vi "Set Log File Producer Flag.vi"(8 "error in":errorcluster, 10 "log file producer":bool, 11 "custom device item in":T1 format="%.0x") -> (0 "error out":errorcluster, 3 "custom device item out":T1 format="%.0x")   [LabVIEW 2027, in "Embedded Data Logger Scripting.lvlib"]
uses:
  Embedded Data Logger Scripting.lvlib
  <vilib>/NI VeriStand/Custom Device API/Custom Device Item Ref.ctl
  <vilib>/NI VeriStand/Custom Device API/Custom Device API.lvlib
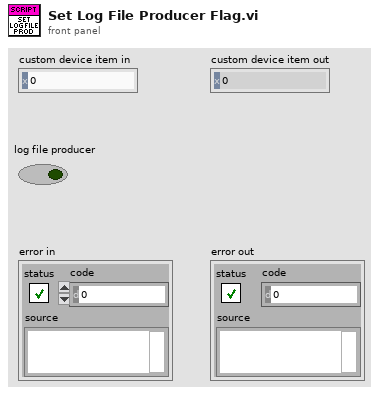
[diagram p1: front panel]
types:
  T1 = typedef "Custom Device API.lvlib/Custom Device Item Ref.ctl" = u64
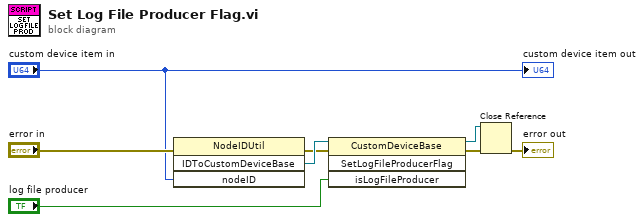
[diagram p0: block diagram]
diagram:
  n1 = invoke class="NodeIDUtil" method="IDToCustomDeviceBase"(error in="error in", "nodeID"="custom device item in") -> (error out=w3:errorcluster, "IDToCustomDeviceBase"=w8:refnum<k39>)  [unwired: 2 in, 2 out]
  n2 = invoke class="CustomDeviceBase" method="SetLogFileProducerFlag"(reference=w8, error in=w3, "isLogFileProducer"="log file producer") -> (reference out=w4:refnum<k39>, error out=w5:errorcluster)  [unwired: 1 in, 2 out]
  n3 = Close Reference(reference=w4, error in (no error)=w5) -> (error out=→"error out":errorcluster)
  "custom device item out" <- "custom device item in"
